vi "SCRIPT_PostCloneTemplate.vi"(9 "Modules Installed":string[](array[string]), 10 "Instance Library":refnum<vi>, 11 "App Ref":refnum<vi>) -> (0 "error out":errorcluster)   [LabVIEW 2020, in "Event Messenger Priority.Scripting.lvlib"]
uses:
  Event Messenger Priority.Scripting.lvlib
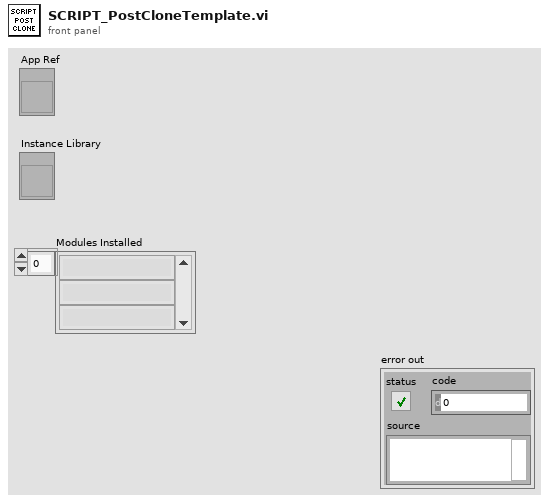
[diagram p1: front panel]
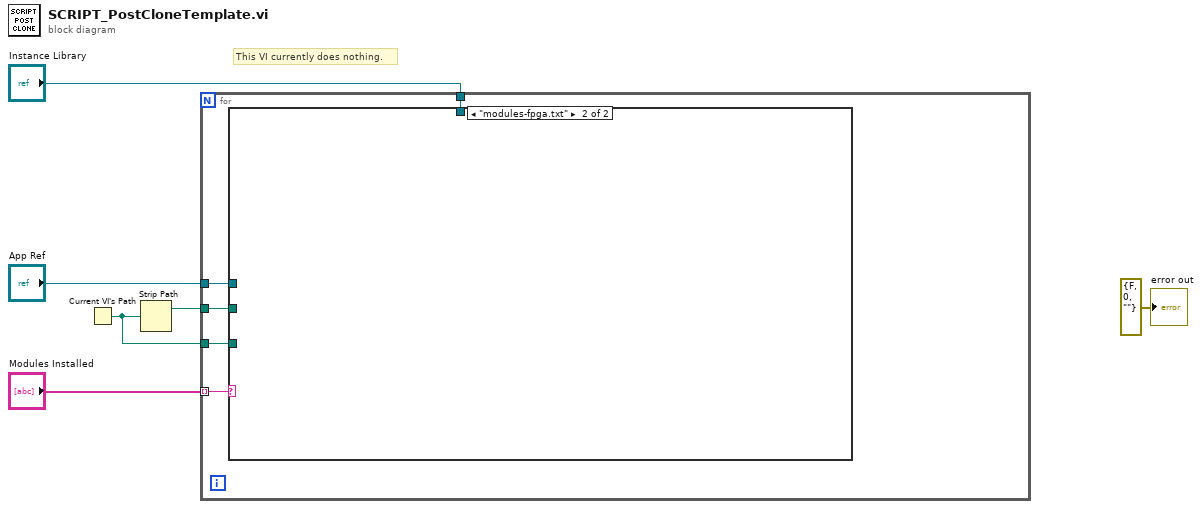
[diagram p0: block diagram]
diagram:
  # "This VI currently does nothing."
  n1 = Current VI's Path() -> (path=w3:path)
  n2 = Strip Path(path=w3) -> (stripped path=w4:path)  [unwired: 1 out]
  n3 = for {
    tunnel: "App Ref" -> [w11]
    tunnel: "Instance Library" -> [w10]
    tunnel: w4 -> [w9]
    tunnel: w3 -> [w8]
    tunnel: "Modules Installed" -> [w7] mode=indexing
    n4 = case shown="\"modules-fpga.txt\"" w7 {
      tunnel: w11 -> [_ _]
      tunnel: w10 -> [_ _]
      tunnel: w9 -> [_ _]
      tunnel: w8 -> [_ _]
      frame Default {
      }
      frame "modules-fpga.txt" {
      }
    }
  }
  "error out" <- errorcluster {"status"=FALSE, "code"=0, "source"=""} ("error out")
